vi "globalstatus.vi"() -> ()   [LabVIEW 2012]
panel:
  in  "status":u16(ring) items=["login", "calibration", "test"]
  out "author":bool
  in  "sample sn":string[](array[string])
  out "tangent":dbl[][](array[numeric])
  out "working":bool[](array[boolean])
  in  "sample port":refnum<visa-resource-name>[](array[refnum])
  in  "do":dbl[](array[numeric])
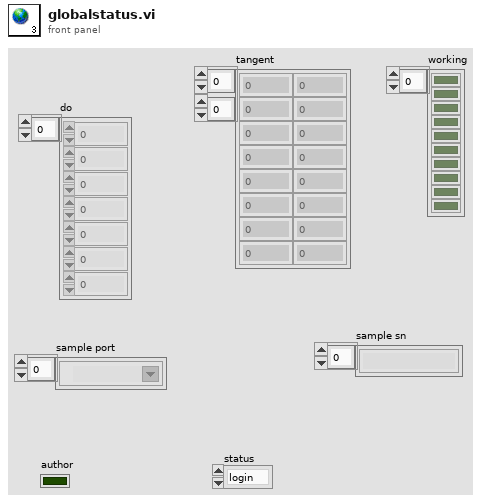
[diagram p1: front panel]
diagram:
